vi "제어기(1215).vi"() -> ()   [LabVIEW 2019]
uses:
  <vilib>/Platform/TimedLoop/XDataNode/timing_clust.ctl
  <vilib>/Platform/TimedLoop/XDataNode/nitl_modes.ctl
  <vilib>/Platform/TimedLoop/XDataNode/wakeup.ctl
  <vilib>/FPGAPlugInAG/myRIO-1900/niLvFpga_Open_myRIO-1900.vi
  <vilib>/rvi/interface/common/dynamic/niFpgaDynamicAddResources.vi
  <vilib>/Utility/error.llb/Error Cluster From Error Code.vi
  <vilib>/rvi/errors/niLvFpgaAdjustHostInterfaceError.vi
  <vilib>/rvi/interface/nirviOpenFPGA/nirviOpenFPGA.xnode
  Encoder_PWM.vi
  <vilib>/rvi/interface/nirviReadWriteControl/nirviReadWriteControl.xnode
  <vilib>/Platform/TimedLoop/XDataNode/XDataNode.xnode
  <vilib>/rvi/interface/Simulation/niFpgaSimulationCallBeginRW.vi
  <vilib>/Platform/TimedLoop/XDataNode/XDNodeRunTimeDep.lvlib
  NiFpgaLv.dll
panel:
  in  "Kp 3":dbl
  in  "Kd 3":dbl
  in  "Ki 3":dbl
  in  "Kp 2":dbl
  in  "Kd 2":dbl
  in  "Ki 2":dbl
  out "u 3":dbl
  out "Mea 3":dbl
  out "e 3":dbl
  out "u 2":dbl
  out "Mea 2":dbl
  out "e 2":dbl
  out "도르래 Ref":dbl=18000.0 format="%#_13g"
  out "오른 바퀴 Ref":dbl=18000.0 format="%#_13g"
  out "왼쪽바퀴 Ref":dbl=18000.0 format="%#_13g"
  out "u":dbl
  out "Mea":dbl
  out "e":dbl
  in  "Ki":dbl
  in  "Kd":dbl
  in  "Kp":dbl
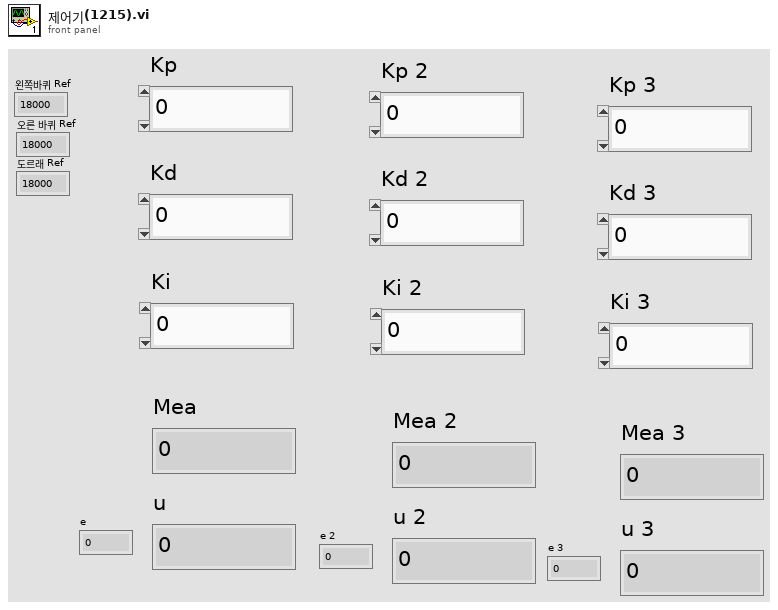
[diagram p1: front panel]
types:
  T1 = typedef "XDNodeRunTimeDep.lvlib/timing_clust.ctl" = cluster{"Expected End [f-1]":u64, "Actual End [f-1]":u64, "Finished Late? [f-1]":bool, "Expected End [i-1]":u64, "Actual End [i-1]":u64, "Finished Late? [i-1]":bool, "Expected Start [i]":u64, "Actual Start [i]":u64, "Expected Start [f]":u64, "Actual Start [f]":u64, "Source Name":string, "Structure Name":string, "Period":i64, "Deadline":i64, "Offset":i64, "Start":i64, "Priority":i32, "Timeout":i32, "Mode":T2, "Wakeup Reason":T3, "Error":errorcluster, "Source Type":string, "Secondary Source Type":string, "Global End Time":u64, "Global Start Time":u64, "Frame Duration":u64, "Iteration Duration":u64, "Assigned CPU":i32, "I/O Scan Engine Mode":u32}
  T2 = typedef "XDNodeRunTimeDep.lvlib/nitl_modes.ctl" = enum32{"No Change", "Process missed periods, maintain original phase", "Discard missed periods, maintain original phase", "Process missed periods, ignore original phase", "Discard missed periods, ignore original phase"}
  T3 = typedef "XDNodeRunTimeDep.lvlib/wakeup.ctl" = enum32{"Normal", "Aborted", "Asynchronous wakeup", "Timing source error", "Timed loop error", "Timeout"}
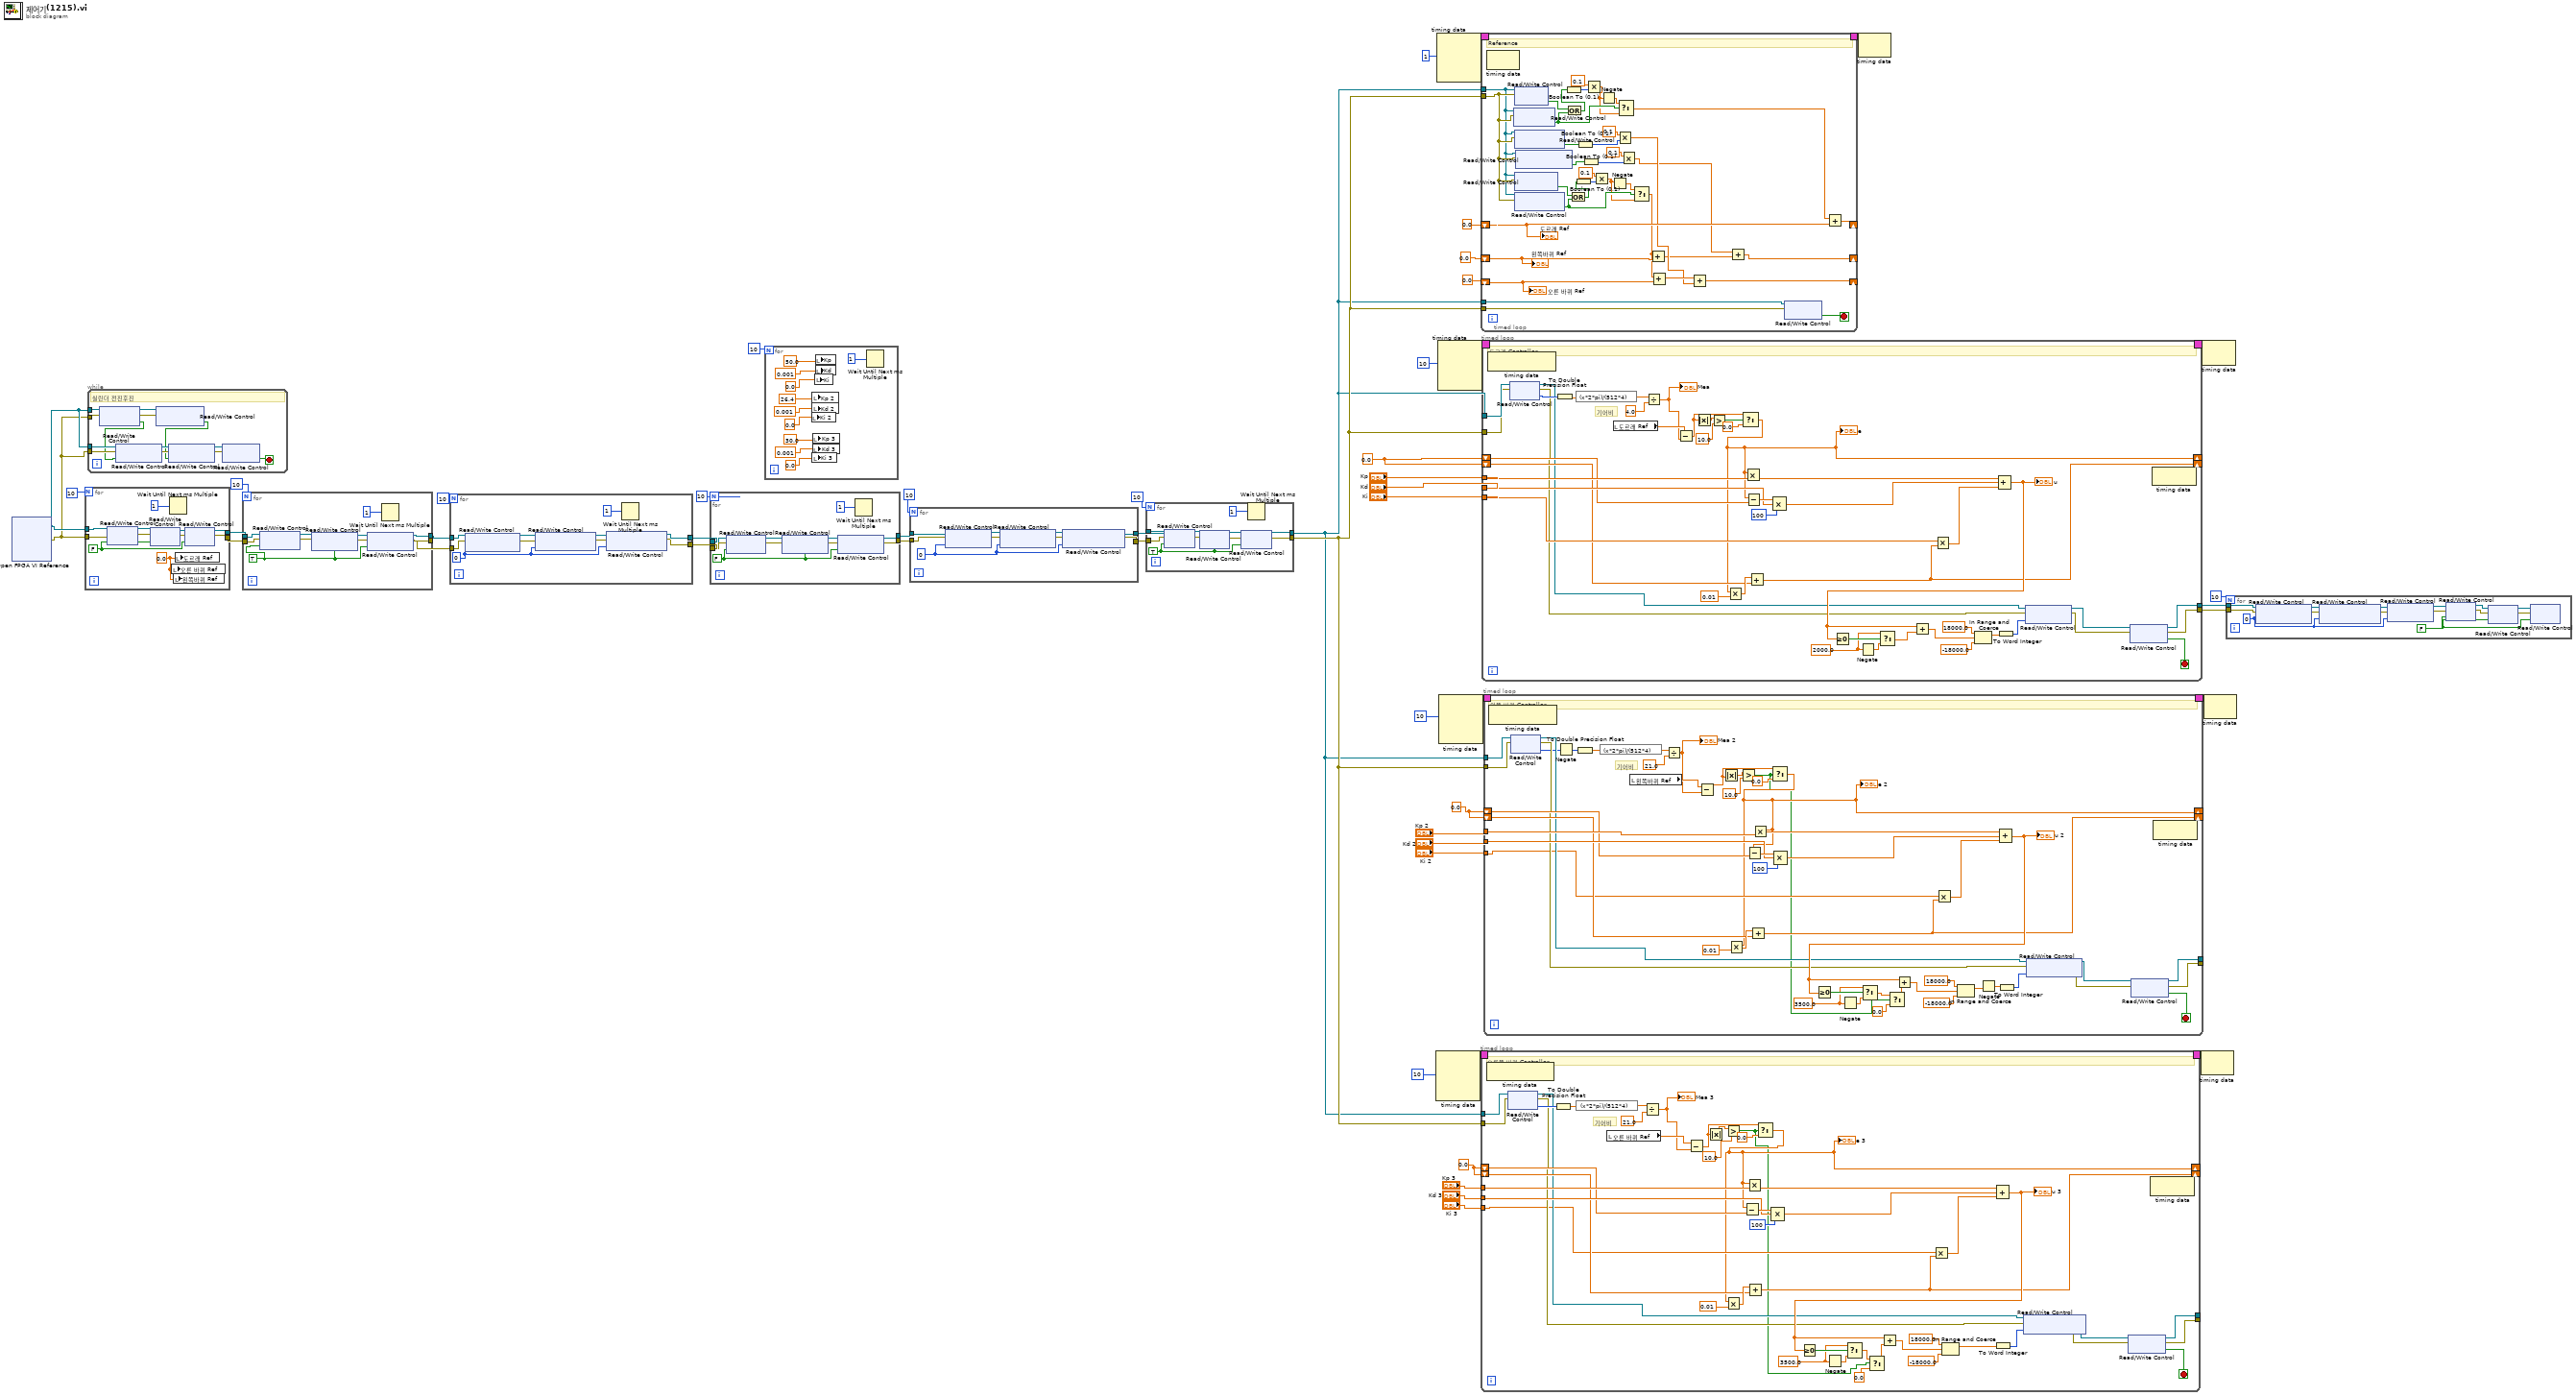
[diagram p0: block diagram]
diagram:
  w3 = 0.0 ("e")
  w4 = 0.0 ("e")
  w33 = 0.0 ("e")
  n1 = xnode "Open FPGA VI Reference"() -> ("FPGA VI Reference Out"=w32:refnum<k20>, "error out"=w31:errorcluster)  [unwired: 2 in]
  n2 = for {
    N: 10 -> [_]
    tunnel: w32 -> [w54]
    tunnel: [w57] -> w47
    tunnel: [w58] -> w46
    tunnel: w31 -> [w53]
    w52 = 0.0 ("Ref")
    w59 = FALSE
    n3 = xnode "Read/Write Control"("FPGA VI Reference In"=w54, "error in"=w53) -> ("FPGA VI Reference Out"=w56:refnum<k20>, "error out"=w55:errorcluster)  [unwired: 1 in]
    n4 = xnode "Read/Write Control"("FPGA VI Reference In"=w56, "error in"=w55, "ena 2"=w59) -> ("FPGA VI Reference Out"=w61:refnum<k20>, "error out"=w60:errorcluster)
    n5 = Wait Until Next ms Multiple(millisecond multiple=1) -> ()  [unwired: 1 out]
    n6 = local write "오른 바퀴 Ref"(w52) -> ()
    n7 = local write "왼쪽바퀴 Ref"(w52) -> ()
    n8 = local write "도르래 Ref"(w52) -> ()
    n9 = xnode "Read/Write Control"("FPGA VI Reference In"=w61, "error in"=w60, "ena 3"=w59) -> ("FPGA VI Reference Out"=w58:refnum<k20>, "error out"=w57:errorcluster)
  }
  n10 = while {
    tunnel: w32 -> [w75]
    tunnel: w31 -> [w74]
    tunnel: w32 -> [w71]
    tunnel: w31 -> [w69]
    stop <- w63 stop-if-true
    # "실린더 전진후진"
    n11 = xnode "Read/Write Control"("FPGA VI Reference In"=w75, "error in"=w74) -> ("FPGA VI Reference Out"=w73:refnum<k20>, "error out"=w72:errorcluster, "왼쪽x왼쪽"=w67:bool)
    n12 = xnode "Read/Write Control"("FPGA VI Reference In"=w71, "error in"=w69, "실린더 전진"=w67) -> ("FPGA VI Reference Out"=w70:refnum<k20>, "error out"=w68:errorcluster)
    n13 = xnode "Read/Write Control"("FPGA VI Reference In"=w73, "error in"=w72) -> ("왼쪽x오른쪽"=w66:bool)  [unwired: 2 out]
    n14 = xnode "Read/Write Control"("FPGA VI Reference In"=w70, "error in"=w68, "실린더 후진"=w66) -> ("FPGA VI Reference Out"=w65:refnum<k20>, "error out"=w64:errorcluster)
    n15 = xnode "Read/Write Control"("FPGA VI Reference In"=w65, "error in"=w64) -> ("비상정지"=w63:bool)  [unwired: 2 out]
  }
  n16 = for {
    N: 10 -> [_]
    tunnel: w47 -> [w77]
    tunnel: w46 -> [w78]
    tunnel: [w84] -> w43
    tunnel: [w83] -> w42
    w76 = TRUE
    n17 = xnode "Read/Write Control"("FPGA VI Reference In"=w78, "error in"=w77, "Enc_Reset"=w76) -> ("FPGA VI Reference Out"=w80:refnum<k20>, "error out"=w79:errorcluster)
    n18 = xnode "Read/Write Control"("FPGA VI Reference In"=w80, "error in"=w79, "Enc_Reset 2"=w76) -> ("FPGA VI Reference Out"=w81:refnum<k20>, "error out"=w82:errorcluster)
    n19 = xnode "Read/Write Control"("FPGA VI Reference In"=w81, "error in"=w82, "Enc_Reset 3"=w76) -> ("FPGA VI Reference Out"=w83:refnum<k20>, "error out"=w84:errorcluster)
    n20 = Wait Until Next ms Multiple(millisecond multiple=1) -> ()  [unwired: 1 out]
  }
  n21 = for {
    N: 10 -> [_]
    tunnel: w43 -> [w90]
    tunnel: w42 -> [w89]
    tunnel: [w91] -> w40
    tunnel: [w92] -> w39
    w86 = 0
    n22 = xnode "Read/Write Control"("FPGA VI Reference In"=w89, "error in"=w90, "Homing Value"=w86) -> ("FPGA VI Reference Out"=w88:refnum<k20>, "error out"=w87:errorcluster)
    n23 = xnode "Read/Write Control"("FPGA VI Reference In"=w88, "error in"=w87, "Homing Value 2"=w86) -> ("FPGA VI Reference Out"=w94:refnum<k20>, "error out"=w93:errorcluster)
    n24 = xnode "Read/Write Control"("FPGA VI Reference In"=w94, "error in"=w93, "Homing Value 3"=w86) -> ("FPGA VI Reference Out"=w92:refnum<k20>, "error out"=w91:errorcluster)
    n25 = Wait Until Next ms Multiple(millisecond multiple=1) -> ()  [unwired: 1 out]
  }
  n26 = for {
    N: 10 -> [_]
    tunnel: w40 -> [w100]
    tunnel: w39 -> [w99]
    tunnel: [w102] -> w28
    tunnel: [w101] -> w29
    w96 = FALSE
    n27 = xnode "Read/Write Control"("FPGA VI Reference In"=w99, "error in"=w100, "Enc_Reset"=w96) -> ("FPGA VI Reference Out"=w97:refnum<k20>, "error out"=w98:errorcluster)
    n28 = xnode "Read/Write Control"("FPGA VI Reference In"=w97, "error in"=w98, "Enc_Reset 2"=w96) -> ("FPGA VI Reference Out"=w104:refnum<k20>, "error out"=w103:errorcluster)
    n29 = xnode "Read/Write Control"("FPGA VI Reference In"=w104, "error in"=w103, "Enc_Reset 3"=w96) -> ("FPGA VI Reference Out"=w101:refnum<k20>, "error out"=w102:errorcluster)
    n30 = Wait Until Next ms Multiple(millisecond multiple=1) -> ()  [unwired: 1 out]
  }
  n31 = for {
    N: 10 -> [_]
    n32 = local write "Ki 2"(0.0 ("e")) -> ()
    n33 = local write "Kp 2"(26.4 ("e")) -> ()
    n34 = local write "Kd 2"(0.001 ("e")) -> ()
    n35 = local write "Ki 3"(0.0 ("e")) -> ()
    n36 = local write "Kp 3"(30.0 ("e")) -> ()
    n37 = local write "Kd 3"(0.001 ("e")) -> ()
    n38 = local write "Ki"(0.0 ("e")) -> ()
    n39 = local write "Kp"(50.0 ("e")) -> ()
    n40 = local write "Kd"(0.001 ("e")) -> ()
    n41 = Wait Until Next ms Multiple(millisecond multiple=1) -> ()  [unwired: 1 out]
  }
  n42 = for {
    N: 10 -> [_]
    tunnel: w29 -> [w117]
    tunnel: w28 -> [w118]
    tunnel: [w122] -> w27
    tunnel: [w121] -> w26
    w116 = 0
    n43 = xnode "Read/Write Control"("FPGA VI Reference In"=w117, "error in"=w118, "도르래 입력"=w116) -> ("FPGA VI Reference Out"=w120:refnum<k20>, "error out"=w119:errorcluster)
    n44 = xnode "Read/Write Control"("FPGA VI Reference In"=w120, "error in"=w119, "왼쪽 바퀴 입력"=w116) -> ("FPGA VI Reference Out"=w124:refnum<k20>, "error out"=w123:errorcluster)
    n45 = xnode "Read/Write Control"("FPGA VI Reference In"=w124, "error in"=w123, "오른쪽 바퀴 입력"=w116) -> ("FPGA VI Reference Out"=w122:refnum<k20>, "error out"=w121:errorcluster)
  }
  n46 = for {
    N: 10 -> [_]
    tunnel: [w131] -> w11
    tunnel: [w130] -> w12
    tunnel: w27 -> [w129]
    tunnel: w26 -> [w128]
    w125 = TRUE
    n47 = xnode "Read/Write Control"("FPGA VI Reference In"=w129, "error in"=w128, "ena"=w125) -> ("FPGA VI Reference Out"=w126:refnum<k20>, "error out"=w127:errorcluster)
    n48 = xnode "Read/Write Control"("FPGA VI Reference In"=w126, "error in"=w127, "ena 2"=w125) -> ("FPGA VI Reference Out"=w132:refnum<k20>, "error out"=w133:errorcluster)
    n49 = xnode "Read/Write Control"("FPGA VI Reference In"=w132, "error in"=w133, "ena 3"=w125) -> ("FPGA VI Reference Out"=w131:refnum<k20>, "error out"=w130:errorcluster)
    n50 = Wait Until Next ms Multiple(millisecond multiple=1) -> ()  [unwired: 1 out]
  }
  n51 = node-c288(i64 10 ("주기")) -> (w17:T1)  [unwired: 3 in]
  n52 = node-c288(i64 1 ("주기")) -> (w51:T1)  [unwired: 3 in]
  n53 = node-c288(i64 10 ("주기")) -> (w49:T1)  [unwired: 3 in]
  n54 = node-c288(i64 10 ("주기")) -> (w19:T1)  [unwired: 3 in]
  n55 = timed-loop {
    timing: w17 -> [_]
    timing-out: [_] -> w16
    tunnel: "Kp 3" -> [w171]
    tunnel: "Kd 3" -> [w170]
    shift-right: [w146] -> _
    shift-left: w3 -> [w169]
    shift-right: [w157] -> _
    shift-left: w3 -> [w168]
    tunnel: w11 -> [w160]
    tunnel: w12 -> [w159]
    tunnel: [w153] -> _
    tunnel: [w152] -> _
    tunnel: "Ki 3" -> [w148]
    stop <- w154 stop-if-true
    w163 = 3500.0
    # "기어비"
    # "오른쪽 바퀴 Controller"
    n56 = node-c288() -> ()  [unwired: 1 in, 1 out]
    n57 = xnode "Read/Write Control"("FPGA VI Reference In"=w160, "error in"=w159) -> ("FPGA VI Reference Out"=w151:refnum<k20>, "error out"=w150:errorcluster, "Enc 3"=w161:i32)
    n58 = To Double Precision Float(number=w161) -> (double precision float=w142:dbl)
    n59 = expression code="(x*2*pi)/(512*4)"(w142) -> (w141:dbl)
    n60 = local read "오른 바퀴 Ref"() -> (w172:dbl)
    n61 = Divide(x=w141, y=21.0) -> (x/y=w149:dbl)
    "Mea 3" <- w149
    n62 = Subtract(x=w172, y=w149) -> (x-y=w145:dbl)
    n63 = Absolute Value(x=w145) -> (abs(x)=w143:dbl)
    n64 = Greater?(x=w143, y=10.0) -> (0:w137:bool)
    n65 = Select(t=w145, s=w137, f=0.0 ("y")) -> (s? t:f=w146:dbl)
    "e 3" <- w146
    n66 = Multiply(x=w146, y=0.01) -> (x*y=w173:dbl)
    n67 = Subtract(x=w146, y=w169) -> (x-y=w178:dbl)
    n68 = Multiply(x=w146, y=w171) -> (x*y=w177:dbl)
    n69 = Add(x=w173, y=w168) -> (x+y=w157:dbl)
    n70 = Compound Arithmetic op=MULTIPLY(w178, w170, 100) -> (w179:dbl)
    n71 = Negate(x=w163) -> (-x=w162:dbl)
    n72 = Multiply(x=w148, y=w157) -> (x*y=w175:dbl)
    n73 = Compound Arithmetic op=ADD(w177, w179, w175) -> (w158:dbl)
    "u 3" <- w158
    n74 = Greater Or Equal To 0?(x=w158) -> (x >= 0?=w164:bool)
    n75 = Select(t=w163, s=w164, f=w162) -> (s? t:f=w136:dbl)
    n76 = Select(t=w136, s=w137, f=0.0) -> (s? t:f=w138:dbl)
    n77 = Add(x=w158, y=w138) -> (x+y=w165:dbl)
    n78 = In Range and Coerce(upper limit=18000.0, x=w165, lower limit=-18000.0) -> (coerced(x)=w139:dbl)  [unwired: 1 out]
    n79 = To Word Integer(number=w139) -> (16bit integer=w140:i16)
    n80 = xnode "Read/Write Control"("FPGA VI Reference In"=w151, "error in"=w150, "오른쪽 바퀴 입력"=w140) -> ("FPGA VI Reference Out"=w155:refnum<k20>, "error out"=w156:errorcluster)
    n81 = xnode "Read/Write Control"("FPGA VI Reference In"=w155, "error in"=w156) -> ("FPGA VI Reference Out"=w152:refnum<k20>, "error out"=w153:errorcluster, "비상정지"=w154:bool)
    n82 = node-c288() -> ()  [unwired: 1 in, 1 out]
  }
  n83 = timed-loop {
    timing: w51 -> [_]
    timing-out: [_] -> w50
    shift-right: [w204] -> _
    shift-left: 0.0 ("y") -> [w209]
    shift-right: [w184] -> _
    shift-left: 0.0 ("y") -> [w210]
    shift-right: [w216] -> _
    shift-left: 0.0 ("y") -> [w215]
    tunnel: w12 -> [w202]
    tunnel: w11 -> [w201]
    tunnel: w12 -> [w200]
    tunnel: w11 -> [w199]
    stop <- w203 stop-if-true
    # "Reference"
    n84 = node-c288() -> ()  [unwired: 1 in, 1 out]
    n85 = xnode "Read/Write Control"("FPGA VI Reference In"=w199, "error in"=w200) -> ("왼쪽Y아래"=w217:bool)  [unwired: 2 out]
    n86 = xnode "Read/Write Control"("FPGA VI Reference In"=w199, "error in"=w200) -> ("왼쪽Y위"=w219:bool)  [unwired: 2 out]
    n87 = xnode "Read/Write Control"("FPGA VI Reference In"=w199, "error in"=w200) -> ("오른쪽X 왼쪽"=w207:bool)  [unwired: 2 out]
    n88 = xnode "Read/Write Control"("FPGA VI Reference In"=w199, "error in"=w200) -> ("오른쪽Y 위"=w211:bool)  [unwired: 2 out]
    n89 = xnode "Read/Write Control"("FPGA VI Reference In"=w199, "error in"=w200) -> ("오른쪽Y 아래"=w212:bool)  [unwired: 2 out]
    n90 = xnode "Read/Write Control"("FPGA VI Reference In"=w199, "error in"=w200) -> ("오른쪽X 오른쪽"=w206:bool)  [unwired: 2 out]
    n91 = Or(x=w219, y=w217) -> (x .or. y?=w218:bool)
    n92 = Boolean To (0,1)(Boolean=w218) -> (0, 1=w196:i16)
    n93 = Or(x=w211, y=w212) -> (x .or. y?=w213:bool)
    n94 = Boolean To (0,1)(Boolean=w213) -> (0, 1=w187:i16)
    n95 = Boolean To (0,1)(Boolean=w207) -> (0, 1=w193:i16)
    n96 = Boolean To (0,1)(Boolean=w206) -> (0, 1=w190:i16)
    n97 = Multiply(x=0.1, y=w196) -> (x*y=w195:dbl)
    n98 = Multiply(x=0.1, y=w187) -> (x*y=w185:dbl)
    n99 = Negate(x=w195) -> (-x=w198:dbl)
    n100 = Negate(x=w185) -> (-x=w197:dbl)
    n101 = Multiply(x=0.1, y=w193) -> (x*y=w192:dbl)
    n102 = Select(t=w198, s=w217, f=w195) -> (s? t:f=w214:dbl)
    n103 = Multiply(x=0.1, y=w190) -> (x*y=w188:dbl)
    n104 = Select(t=w197, s=w212, f=w185) -> (s? t:f=w208:dbl)
    n105 = Add(x=w208, y=w209) -> (x+y=w183:dbl)
    n106 = Add(x=w208, y=w210) -> (x+y=w205:dbl)
    n107 = Add(x=w205, y=w192) -> (x+y=w184:dbl)
    n108 = Add(x=w188, y=w183) -> (x+y=w204:dbl)
    n109 = xnode "Read/Write Control"("FPGA VI Reference In"=w201, "error in"=w202) -> ("비상정지"=w203:bool)  [unwired: 2 out]
    n110 = Add(x=w214, y=w215) -> (x+y=w216:dbl)
    "왼쪽바퀴 Ref" <- w209
    "오른 바퀴 Ref" <- w210
    "도르래 Ref" <- w215
  }
  n111 = timed-loop {
    timing: w49 -> [_]
    timing-out: [_] -> w48
    tunnel: "Kp" -> [w254]
    tunnel: "Kd" -> [w253]
    tunnel: "Ki" -> [w252]
    shift-right: [w225] -> _
    shift-left: w33 -> [w251]
    shift-right: [w236] -> _
    shift-left: w33 -> [w250]
    tunnel: w11 -> [w240]
    tunnel: w12 -> [w239]
    tunnel: [w232] -> w24
    tunnel: [w231] -> w23
    stop <- w233 stop-if-true
    w244 = 2000.0
    # "기어비"
    # "도르래 Controller"
    n112 = node-c288() -> ()  [unwired: 1 in, 1 out]
    n113 = xnode "Read/Write Control"("FPGA VI Reference In"=w240, "error in"=w239) -> ("FPGA VI Reference Out"=w230:refnum<k20>, "error out"=w229:errorcluster, "Enc"=w241:i32)
    n114 = To Double Precision Float(number=w241) -> (double precision float=w263:dbl)
    n115 = expression code="(x*2*pi)/(512*4)"(w263) -> (w265:dbl)
    n116 = local read "도르래 Ref"() -> (w255:dbl)
    n117 = Divide(x=w265, y=4.0) -> (x/y=w228:dbl)
    "Mea" <- w228
    n118 = Subtract(x=w255, y=w228) -> (x-y=w223:dbl)
    n119 = Absolute Value(x=w223) -> (abs(x)=w224:dbl)
    n120 = Greater?(x=w224, y=10.0) -> (0:w227:bool)
    n121 = Select(t=w223, s=w227, f=0.0 ("y")) -> (s? t:f=w225:dbl)
    "e" <- w225
    n122 = Multiply(x=w225, y=0.01) -> (x*y=w256:dbl)
    n123 = Multiply(x=w225, y=w254) -> (x*y=w260:dbl)
    n124 = Subtract(x=w225, y=w251) -> (x-y=w261:dbl)
    n125 = Add(x=w256, y=w250) -> (x+y=w236:dbl)
    n126 = Compound Arithmetic op=MULTIPLY(w261, w253, 100) -> (w262:dbl)
    n127 = Negate(x=w244) -> (-x=w243:dbl)
    n128 = Multiply(x=w252, y=w236) -> (x*y=w258:dbl)
    n129 = Compound Arithmetic op=ADD(w260, w262, w258) -> (w237:dbl)
    "u" <- w237
    n130 = Greater Or Equal To 0?(x=w237) -> (x >= 0?=w245:bool)
    n131 = Select(t=w244, s=w245, f=w243) -> (s? t:f=w242:dbl)
    n132 = Add(x=w237, y=w242) -> (x+y=w246:dbl)
    n133 = In Range and Coerce(upper limit=18000.0, x=w246, lower limit=-18000.0) -> (coerced(x)=w249:dbl)  [unwired: 1 out]
    n134 = To Word Integer(number=w249) -> (16bit integer=w238:i16)
    n135 = xnode "Read/Write Control"("FPGA VI Reference In"=w230, "error in"=w229, "도르래 입력"=w238) -> ("FPGA VI Reference Out"=w234:refnum<k20>, "error out"=w235:errorcluster)
    n136 = xnode "Read/Write Control"("FPGA VI Reference In"=w234, "error in"=w235) -> ("FPGA VI Reference Out"=w231:refnum<k20>, "error out"=w232:errorcluster, "비상정지"=w233:bool)
    n137 = node-c288() -> ()  [unwired: 1 in, 1 out]
  }
  n138 = timed-loop {
    timing: w19 -> [_]
    timing-out: [_] -> w18
    tunnel: "Kp 2" -> [w306]
    tunnel: "Kd 2" -> [w305]
    shift-right: [w282] -> _
    shift-left: w4 -> [w304]
    shift-right: [w292] -> _
    shift-left: w4 -> [w303]
    tunnel: w11 -> [w296]
    tunnel: w12 -> [w295]
    tunnel: [w288] -> _
    tunnel: [w287] -> _
    tunnel: "Ki 2" -> [w283]
    stop <- w289 stop-if-true
    w298 = 3500.0
    # "기어비"
    # "왼쪽 바퀴 Controller"
    n139 = node-c288() -> ()  [unwired: 1 in, 1 out]
    n140 = xnode "Read/Write Control"("FPGA VI Reference In"=w296, "error in"=w295) -> ("FPGA VI Reference Out"=w286:refnum<k20>, "error out"=w285:errorcluster, "Enc 2"=w272:i32)
    n141 = Negate(x=w272) -> (-x=w273:i32)
    n142 = To Double Precision Float(number=w273) -> (double precision float=w276:dbl)
    n143 = expression code="(x*2*pi)/(512*4)"(w276) -> (w277:dbl)
    n144 = local read "왼쪽바퀴 Ref"() -> (w307:dbl)
    n145 = Divide(x=w277, y=21.0) -> (x/y=w284:dbl)
    "Mea 2" <- w284
    n146 = Subtract(x=w307, y=w284) -> (x-y=w280:dbl)
    n147 = Absolute Value(x=w280) -> (abs(x)=w279:dbl)
    n148 = Greater?(x=w279, y=10.0) -> (0:w270:bool)
    n149 = Select(t=w280, s=w270, f=0.0 ("y")) -> (s? t:f=w282:dbl)
    "e 2" <- w282
    n150 = Multiply(x=w282, y=0.01) -> (x*y=w308:dbl)
    n151 = Subtract(x=w282, y=w304) -> (x-y=w313:dbl)
    n152 = Add(x=w308, y=w303) -> (x+y=w292:dbl)
    n153 = Multiply(x=w282, y=w306) -> (x*y=w312:dbl)
    n154 = Compound Arithmetic op=MULTIPLY(w313, w305, 100) -> (w314:dbl)
    n155 = Negate(x=w298) -> (-x=w297:dbl)
    n156 = Multiply(x=w283, y=w292) -> (x*y=w310:dbl)
    n157 = Compound Arithmetic op=ADD(w312, w314, w310) -> (w293:dbl)
    "u 2" <- w293
    n158 = Greater Or Equal To 0?(x=w293) -> (x >= 0?=w299:bool)
    n159 = Select(t=w298, s=w299, f=w297) -> (s? t:f=w268:dbl)
    n160 = Select(t=w268, s=w270, f=0.0) -> (s? t:f=w271:dbl)
    n161 = Add(x=w293, y=w271) -> (x+y=w300:dbl)
    n162 = In Range and Coerce(upper limit=18000.0, x=w300, lower limit=-18000.0) -> (coerced(x)=w274:dbl)  [unwired: 1 out]
    n163 = Negate(x=w274) -> (-x=w275:dbl)
    n164 = To Word Integer(number=w275) -> (16bit integer=w294:i16)
    n165 = xnode "Read/Write Control"("FPGA VI Reference In"=w286, "error in"=w285, "왼쪽 바퀴 입력"=w294) -> ("FPGA VI Reference Out"=w290:refnum<k20>, "error out"=w291:errorcluster)
    n166 = xnode "Read/Write Control"("FPGA VI Reference In"=w290, "error in"=w291) -> ("FPGA VI Reference Out"=w287:refnum<k20>, "error out"=w288:errorcluster, "비상정지"=w289:bool)
    n167 = node-c288() -> ()  [unwired: 1 in, 1 out]
  }
  n168 = node-c288(w50) -> ()  [unwired: 1 out]
  n169 = node-c288(w16) -> ()  [unwired: 1 out]
  n170 = node-c288(w48) -> ()  [unwired: 1 out]
  n171 = node-c288(w18) -> ()  [unwired: 1 out]
  n172 = for {
    N: 10 -> [_]
    tunnel: w24 -> [w331]
    tunnel: w23 -> [w330]
    w318 = FALSE
    w323 = i16 0 ("Input")
    n173 = xnode "Read/Write Control"("FPGA VI Reference In"=w330, "error in"=w331, "왼쪽 바퀴 입력"=w323) -> ("FPGA VI Reference Out"=w329:refnum<k20>, "error out"=w328:errorcluster)
    n174 = xnode "Read/Write Control"("FPGA VI Reference In"=w329, "error in"=w328, "오른쪽 바퀴 입력"=w323) -> ("FPGA VI Reference Out"=w325:refnum<k20>, "error out"=w324:errorcluster)
    n175 = xnode "Read/Write Control"("FPGA VI Reference In"=w325, "error in"=w324, "도르래 입력"=w323) -> ("FPGA VI Reference Out"=w321:refnum<k20>, "error out"=w322:errorcluster)
    n176 = xnode "Read/Write Control"("FPGA VI Reference In"=w321, "error in"=w322, "ena"=w318) -> ("FPGA VI Reference Out"=w319:refnum<k20>, "error out"=w320:errorcluster)
    n177 = xnode "Read/Write Control"("FPGA VI Reference In"=w319, "error in"=w320, "ena 2"=w318) -> ("FPGA VI Reference Out"=w326:refnum<k20>, "error out"=w327:errorcluster)
    n178 = xnode "Read/Write Control"("FPGA VI Reference In"=w326, "error in"=w327, "ena 3"=w318) -> ()  [unwired: 2 out]
  }
